vi "Init Actor Core.vi"(8 "error in (no error)":errorcluster, 11 "Measure Object in":refnum<class "Application Controller.lvclass">) -> (0 "error out":errorcluster, 3 "Measure Object out":refnum<class "Application Controller.lvclass">)   [LabVIEW 2018, in "Application Controller.lvclass"]
uses:
  Application Controller.lvclass
  C:/github/LabActor/Template Module/Template Module.lvclass
  C:/Program Files/National Instruments/LabVIEW 2018/vi.lib/ActorFramework/Actor/Actor.lvclass
  Application Controller.lvclass/Application Controller.ctl
  Template Module/Template Module.lvclass/Template Module.ctl
  <vilib>/ActorFramework/Actor/Actor.lvclass/Actor.ctl
  <vilib>/ActorFramework/Message Enqueuer/Message Enqueuer.lvclass/Message Enqueuer.ctl
  Read Launch Notifier.vi
  Template Module/Read Name.vi
  Read Start-up configuration file.vi
  <vilib>/ActorFramework/Message Enqueuer/Init from Existing Queue.vi
  <vilib>/ActorFramework/Message Enqueuer/Enqueue.vi
  Comms/Communications Messages/Init Comms Msg/Init Comms Msg.lvclass
  C:/Program Files/National Instruments/LabVIEW 2018/vi.lib/ActorFramework/Message/Message.lvclass
  Application Controller Messages/Load Complete Msg/Load Complete Msg.lvclass
  <vilib>/ActorFramework/Message Priority Queue/Priority Enqueue.vi
  <vilib>/ActorFramework/Message Enqueuer/Message Enqueuer.lvclass
  Process Controller/Process Controller.lvclass
  <vilib>/ActorFramework/Actor/Actor.lvclass
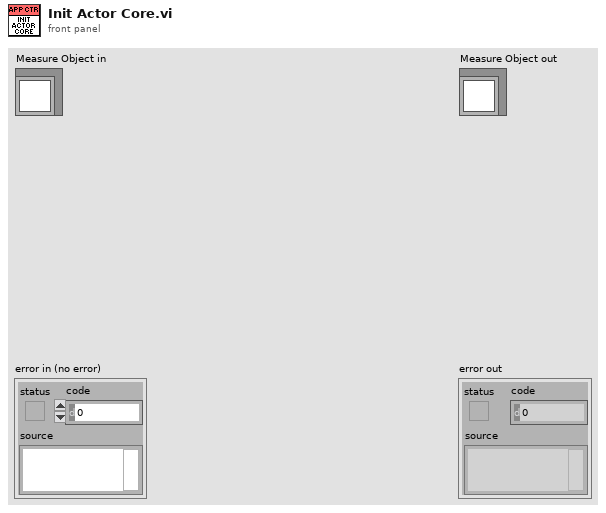
[diagram p1: front panel]
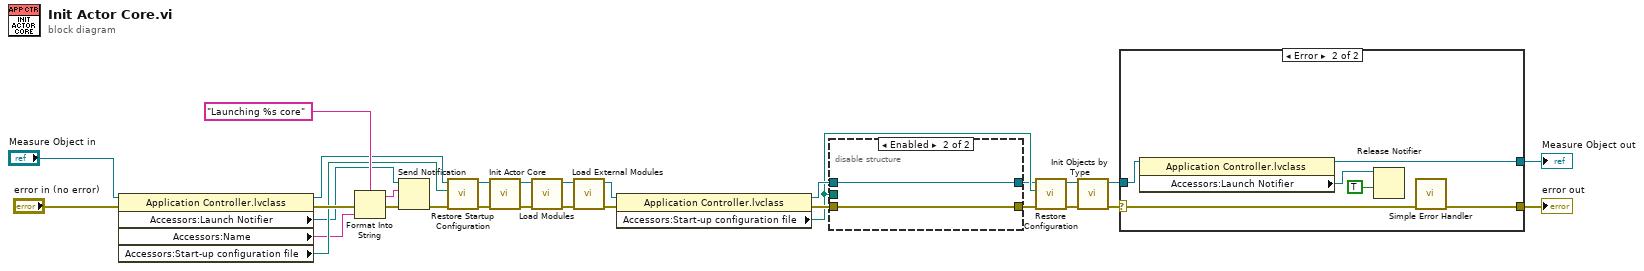
[diagram p0: block diagram]
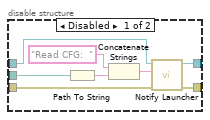
[diagram p2: hidden frame]
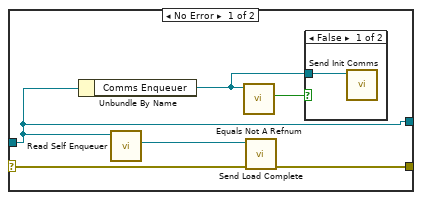
[diagram p3: hidden frame]
diagram:
  n1 = property class="Application Controller.lvclass"(reference="Measure Object in", error in="error in (no error)") -> (reference out=w25:refnum<class "Application Controller.lvclass">, error out=w27:errorcluster, "Accessors:Launch Notifier"=w17:refnum<notifier>, "Accessors:Name"=w18:string, "Accessors:Start-up configuration file"=w19:path)
  n2 = Format Into String(format string="Launching %s core" ("notification"), error in=w27, w18) -> (resulting string=w16:string, error out=w26:errorcluster)  [unwired: 1 in]
  n3 = Send Notification(notification=w16, notifier=w17, error in (no error)=w26) -> (error out=w24:errorcluster)  [unwired: 1 out]
  n4 = call-dynamic "Restore Startup Configuration.vi"("error in (no error)"=w24, "Startup Configuration File"=w19, "Monitor-Pulse in"=w25) -> ("error out"=w23:errorcluster, "Monitor-Pulse out"=w20:refnum<class "Application Controller.lvclass">)  [unwired: 6 in, 1 out]
  n5 = call-parent "Init Actor Core.vi"("error in (no error)"=w23, "Measure Object in"=w20) -> ("error out"=w22:errorcluster, "Measure Object out"=w15:refnum<class "Application Controller.lvclass">)  [unwired: 8 in]
  n6 = call-dynamic "Load Modules.vi"("error in (no error)"=w22, "Application Controller in"=w15) -> ("error out"=w12:errorcluster, "Application Controller out"=w11:refnum<class "Application Controller.lvclass">)  [unwired: 8 in]
  n7 = call-dynamic "Load External Modules.vi"("error in (no error)"=w12, "Application Controller in"=w11) -> ("error out"=w10:errorcluster, "Application Controller out"=w9:refnum<class "Application Controller.lvclass">)  [unwired: 8 in]
  n8 = property class="Application Controller.lvclass"(reference=w9, error in=w10) -> (reference out=w5:refnum<class "Application Controller.lvclass">, error out=w4:errorcluster, "Accessors:Start-up configuration file"=w3:path)
  n9 = disable-structure shown="Enabled" {
    disable-tunnel: w5 -> [w38 w40]
    disable-tunnel: w4 -> [w37 w39]
    disable-tunnel: w3 -> [w35 _]
    disable-tunnel: [w32 w40] -> w2
    disable-tunnel: [w31 w39] -> w1
    frame Disabled {
      n10 = Path To String(path=w35) -> (string=w36:string)
      n11 = Concatenate Strings("Read CFG:  " ("notification"), w36) -> (w33:string)
      n12 = call-dynamic "Notify Launcher.vi"("error in (no error)"=w37, "Notification"=w33, "Application Controller in"=w38) -> ("error out"=w31:errorcluster, "Application Controller out"=w32:refnum<class "Application Controller.lvclass">)  [unwired: 7 in]
    }
    frame Enabled {
    }
  }
  n13 = call-dynamic "Restore Configuration.vi"("error in (no error)"=w1, "File path"=w3, "Measure Object in"=w2) -> ("error out"=w14:errorcluster, "Measure Object out"=w13:refnum<class "Application Controller.lvclass">)  [unwired: 5 in, 2 out]
  n14 = call-dynamic "Init Objects by Type.vi"("error in (no error)"=w14, "Application Controller in"=w13) -> ("error out"=w8:errorcluster, "Application Controller out"=w7:refnum<class "Application Controller.lvclass">)  [unwired: 8 in]
  n15 = case shown="Error" w8 {
    selector: w8 -> [w42 w51]
    tunnel: [w45 w48] -> w21
    tunnel: w7 -> [w41 w53]
    tunnel: [w41 w52] -> w6
    frame No Error {
      n16 = Unbundle By Name(w41) -> ("Comms Enqueuer"=w44:refnum<class "Message Enqueuer.lvclass">)
      n17 = call <vilib>:"Read Self Enqueuer.vi"("Actor"=w41) -> ("Self Enqueuer"=w46:refnum<class "Message Enqueuer.lvclass">)  [unwired: 10 in]
      n18 = call <vilib>:"Equals Not A Refnum.vi"("Message Enqueuer"=w44) -> ("Not a refnum?"=w43:bool)  [unwired: 10 in]
      n19 = call "Send Load Complete.vi"("error in (no error)"=w42, "Message Enqueuer"=w46) -> ("error out"=w45:errorcluster)  [unwired: 8 in, 1 out]
      n20 = case shown="False" w43 {
        tunnel: w44 -> [w47 _]
        frame False {
          n21 = call "Send Init Comms.vi"("Message Enqueuer"=w47) -> ()  [unwired: 9 in, 2 out]
        }
        frame True {
        }
      }
    }
    frame Error {
      n22 = property class="Application Controller.lvclass"(reference=w53) -> (reference out=w52:refnum<class "Application Controller.lvclass">, "Accessors:Launch Notifier"=w49:refnum<notifier>)  [unwired: 1 in, 1 out]
      n23 = Release Notifier(notifier=w49, force destroy? (F)=TRUE) -> ()  [unwired: 1 in, 3 out]
      n24 = call <vilib>:"Simple Error Handler.vi"("error in (no error)"=w51) -> ("error out"=w48:errorcluster)  [unwired: 4 in, 4 out]
    }
  }
  "error out" <- w21
  "Measure Object out" <- w6
